vi "WS1050 16 DUT VSA-CV Sweep HD_Cycling_Ver1.3a.vi"() -> ()   [LabVIEW 2012]
uses:
  WS_VCAP Driver 024/Source/WSVCAP Shell/Type Defs/WSVCAP SHL I2C DUT Mask Mode Enum.ctl
  <vilib>/Utility/file.llb/Read From Spreadsheet File (DBL).vi
panel:
  out "VISA resource name out":refnum<visa-resource-name>="GPIB0::3::INSTR"
  out "date string":string="5/19/2014"
  out "PS1 Out":refnum<visa-resource-name>
  out "Ke2000 Out":refnum<visa-resource-name>="GPIB0::9::INSTR"
  in  "Tab Control":enum32{"Inst Control", "Data Output", "Graphs"}(tab)
  in  "Bank to HD":u16(ring)=5 items=["All OFF", "All ON", "Bank_C1", "Bank_C2", "Bank_C3", "F12+B1", "B1"]
  out "AD7747 Values":string[][](table)
  in  "Lot#":string="4NEMB"
  in  "Wafer#":string="20-EB"
  in  "File Name":string="HD_4NEMB_25_EB_65C_44V_100DC_BRD2_150916_1"
  in  "TMN DC\\CAP Data Log File Path":path=path "C:/WS1050 16 DUT Data"
  in  "SN":string[](array[string])=["1", "2", "3", "4", "5", "6", "7", "8", "9", "10", "11", "12", "13", "14", "15", "16"]
  in  "Test Program":string="WS1050 16 DUT VSA_CV Sweep HD_Cycling Ver1.3a"
  out "Current Date":string="8/28/2014"
  out "Current Time":string="0950"
  in  "Start Date":string="4/24/2014"
  in  "Start Time":string="1542"
  in  "Comment":string="CV Sweep"
  in  "OK Button":bool
  in  "Calibration":bool
  in  "Control Setting":bool
  in  "CP Setting":i32(ring) items=["CP OFF", "CP ON", "CP 35V", "CP 40V", "CP 44V", "CP 50V", "DVA OFF", "DVA ON", "Reg1 ON", "Reg1 OFF", "Reg2 ON", "Reg2 OFF", "Reg3 ON", "Reg3 OFF"]
  in  "VDD(V)":dbl=3.3 format="%.3g"
  in  "Meas Clock Rate (Hz)":dbl=1000000.0 caption="Meas Speed" format="%.1p Hz"
  out "AR  Measurent(Hz)":dbl
  in  "PS1 Source":refnum<visa-resource-name>="GPIB0::5::INSTR"
  in  "Ke2000":refnum<visa-resource-name>="GPIB0::9::INSTR"
  out "Simulate FPGA":bool
  out "Online":bool
  in  "Ke2400":refnum<visa-resource-name>="GPIB0::3::INSTR"
  in  "Initialize AD7747":bool
  in  "DUT Mask Mode":T1=enum."All"
  in  "RFFE Slave Address":u8=7 caption="Slave Address" format="0x%02x"
  out "Activity Log":string="05/19/2014 -- 12:24:35.853::WSVCAP::APP::Application Started\n05/19/2014 -- 12:24:37.606::WSVCAP::WSVCAP SHL::WR I2C-REG:0x0A;MASK:0xFFFFFFFFFFFF;C1 DATA:22:22:22:22:22:22:22:22:22:22:22:22:22:22:22:22;C2 DATA:22:22:22:22:22:22:22:22:22:22:22:22:22:22:22:22;C3 DATA:22:22:22:22:22:22:22:22:22:22:22:22:22:22:22:22\r\n05/19/2014 -- 12:24:37.773::WSVCAP::WSVCAP SHL::WR I2C-ST:0,0,4,1\r\n05/19/2014 -- 12:24:37.903::WSVCAP::WSVCAP SHL::RD I2C-BYTES:4;ADD:0x00;MASK:0xFFFFFFFFFFFF\r\n05/19/2014 -- 12:24:38.045::WSVCAP::WSVCAP SHL::RD I2C:C1 DATA:2:2:2:2:2:2:2:2:2:2:2:2:2:2:2:2|A7:A9:AA:82:82:7F:82:81:82:81:83:82:81:82:82:81|46:36:BB:88:44:A3:E9:2B:32:20:ED:25:BB:3D:68:B|2C:6A:EB:A7:22:56:FE:CC:36:82:D7:B0:3B:48:F9:CC;C2 DATA:2:2:2:2:2:2:2:2:2:2:2:2:2:2:2:2|94:94:94:80:80:80:80:80:81:7E:7E:81:80:7E:80:80|47:33:15:82:62:B:E8:1C:D7:C3:7D:41:7C:B7:4C:2A|C4:B4:AE:8:1E:D1:4E:37:11:C0:6F:63:42:9D:63:B5;C3 DATA:2:2:2:2:2:2:2:2:2:2:2:2:2:2:2:2|95:95:95:81:81:7E:81:80:84:7D:80:83:81:7E:7F:80|AB:C4:14:B5:7B:52:DF:C9:79:5D:5F:30:99:31:1E:F4|6E:5C:F7:A8:C3:EB:7B:EF:33:92:89:77:4D:67:75:DD;STATUS:0:0:4:0\r\n05/19/2014 -- 12:24:38.046::WSVCAP::WSVCAP SHL::WR I2C-REG:0x0A;MASK:0xFFFFFFFFFFFF;C1 DATA:22:22:22:22:22:22:22:22:22:22:22:22:22:22:22:22;C2 DATA:22:22:22:22:22:22:22:22:22:22:22:22:22:22:22:22;C3 DATA:22:22:22:22:22:22:22:22:22:22:22:22:22:22:22:22\r\n05/19/2014 -- 12:24:38.089::WSVCAP::WSVCAP SHL::WR I2C-ST:0,0,4,1\r\n05/19/2014 -- 12:24:38.219::WSVCAP::WSVCAP SHL::RD I2C-BYTES:4;ADD:0x00;MASK:0xFFFFFFFFFFFF\r\n05/19/2014 -- 12:24:38.362::WSVCAP::WSVCAP SHL::RD I2C:C1 DATA:2:2:2:2:2:2:2:2:2:2:2:2:2:2:2:2|A7:AB:AA:82:82:82:83:83:82:82:82:82:7F:82:82:81|4B:32:96:83:3E:61:43:17:25:62:AB:4D:A2:40:2E:5|3C:76:2B:B4:EE:E4:A9:1A:AA:A:26:C7:21:2E:87:5B;C2 DATA:2:2:2:2:2:2:2:2:2:2:2:2:2:2:2:2|94:94:94:80:80:80:80:80:80:7F:80:81:80:80:7F:80|4A:32:19:7D:19:6C:79:46:61:7F:4B:B8:A5:30:F3:14|B4:70:A:8C:9C:DC:43:FA:1E:A:C6:21:A:A9:13:F3;C3 DATA:2:2:2:2:2:2:2:2:2:2:2:2:2:2:2:2|95:97:94:81:80:81:82:81:80:7E:81:84:7F:81:80:80|B2:32:D0:A7:9E:4C:AB:D4:EE:D9:F0:82:B7:91:7:FF|C1:91:B6:3D:D8:E:1B:4F:9F:6A:F1:6C:E7:3F:7:BA;STATUS:0:0:4:0\r\n05/19/2014 -- 12:24:38.364::WSVCAP::WSVCAP SHL::WR I2C-REG:0x0A;MASK:0xFFFFFFFFFFFF;C1 DATA:22:22:22:22:22:22:22:22:22:22:22:22:22:22:22:22;C2 DATA:22:22:22:22:22:22:22:22:22:22:22:22:22:22:22:22;C3 DATA:22:22:22:22:22:22:22:22:22:22:22:22:22:22:22:22\r\n05/19/2014 -- 12:24:38.406::WSVCAP::WSVCAP SHL::WR I2C-ST:0,0,4,1\r\n05/19/2014 -- 12:24:38.536::WSVCAP::WSVCAP SHL::RD I2C-BYTES:4;ADD:0x00;MASK:0xFFFFFFFFFFFF\r\n05/19/2014 -- 12:24:38.678::WSVCAP::WSVCAP SHL::RD I2C:C1 DATA:2:2:2:2:2:2:2:2:2:2:2:2:2:2:2:2|A7:A9:AB:82:82:81:82:82:82:82:82:82:82:82:82:81|46:71:4C:87:43:3D:7F:FC:25:4F:8E:54:97:3E:60:8C|AA:F4:1F:B5:CE:43:1F:36:9:87:9C:78:86:5:B6:8E;C2 DATA:2:2:2:2:2:2:2:2:2:2:2:2:2:2:2:2|94:94:94:80:7F:7F:80:80:80:80:80:81:80:80:80:80|49:36:18:7D:6E:C5:E4:3C:81:2E:41:D3:75:71:E3:72|E8:D3:E6:D1:E0:48:AE:D4:54:D:E8:8E:B4:41:68:4;C3 DATA:2:2:2:2:2:2:2:2:2:2:2:2:2:2:2:2|95:95:95:81:7F:7F:81:81:81:81:81:84:81:81:82:81|B3:F5:90:AB:82:69:7B:93:D0:77:E8:D5:E8:8C:84:E8|B9:AC:EE:2B:B6:71:8F:4A:74:31:56:BB:8A:B7:A0:C8;STATUS:0:0:4:0\r\n05/19/2014 -- 12:24:38.681::WSVCAP::WSVCAP SHL::WR I2C-REG:0x0A;MASK:0xFFFFFFFFFFFF;C1 DATA:22:22:22:22:22:22:22:22:22:22:22:22:22:22:22:22;C2 DATA:22:22:22:22:22:22:22:22:22:22:22:22:22:22:22:22;C3 DATA:22:22:22:22:22:22:22:22:22:22:22:22:22:22:22:22\r\n05/19/2014 -- 12:24:38.723::WSVCAP::WSVCAP SHL::WR I2C-ST:0,0,4,1\r\n05/19/2014 -- 12:24:38.854::WSVCAP::WSVCAP SHL::RD I2C-BYTES:4;ADD:0x00;MASK:0xFFFFFFFFFFFF\r\n05/19/2014 -- 12:24:38.996::WSVCAP::WSVCAP SHL::RD I2C:C1 DATA:2:2:2:2:2:2:2:2:2:2:2:2:2:2:2:2|A7:A9:AA:82:82:7F:83:81:82:81:84:82:7F:82:7F:82|43:FB:E:7F:3C:AD:35:35:26:A2:6C:21:4B:3D:8:6|63:9A:E1:F3:95:32:91:42:90:3C:78:1F:5C:D7:5F:D8;C2 DATA:2:2:2:2:2:2:2:2:2:2:2:2:2:2:2:2|94:94:94:80:80:80:80:80:81:80:7E:81:80:7E:7F:80|48:36:18:7F:5E:3D:69:83:DE:AE:A1:9E:31:AE:BB:96|15:A0:44:17:13:FD:CC:C8:6D:B2:EF:A7:C:C7:3B:F;C3 DATA:2:2:2:2:2:2:2:2:2:2:2:2:2:2:2:2|95:96:94:81:81:7E:82:80:84:80:80:84:7F:7E:7D:82|AD:3B:6D:A9:7C:57:9D:F5:7A:96:23:5C:36:2D:ED:5A|CD:46:DB:3B:C7:BD:70:60:33:B8:B:F7:63:A:51:4D;STATUS:0:0:4:0\r\n05/19/2014 -- 12:24:38.998::WSVCAP::WSVCAP SHL::WR I2C-REG:0x0A;MASK:0xFFFFFFFFFFFF;C1 DATA:22:22:22:22:22:22:22:22:22:22:22:22:22:22:22:22;C2 DATA:22:22:22:22:22:22:22:22:22:22:22:22:22:22:22:22;C3 DATA:22:22:22:22:22:22:22:22:22:22:22:22:22:22:22:22\r\n05/19/2014 -- 12:24:39.040::WSVCAP::WSVCAP SHL::WR I2C-ST:0,0,4,1\r\n05/19/2014 -- 12:24:39.170::WSVCAP::WSVCAP SHL::RD I2C-BYTES:4;ADD:0x00;MASK:0xFFFFFFFFFFFF\r\n05/19/2014 -- 12:24:39.311::WSVCAP::WSVCAP SHL::RD I2C:C1 DATA:2:2:2:2:2:2:2:2:2:2:2:2:2:2:2:2|A7:AA:AB:82:82:81:82:81:82:81:82:82:82:82:7F:82|44:F1:90:87:45:44:C8:2C:2C:F1:FC:1B:94:3B:3C:75|4A:49:95:19:99:73:64:3:23:24:F3:A2:5E:7F:C4:B6;C2 DATA:2:2:2:2:2:2:2:2:2:2:2:2:2:2:2:2|94:94:94:80:80:80:80:7F:80:80:7E:80:80:7E:7F:80|4C:36:17:7D:A8:9F:DE:C7:53:6D:8A:F4:41:A5:C6:E0|90:2E:24:C:D9:22:E4:76:3B:40:1D:53:33:B1:3E:4D;C3 DATA:2:2:2:2:2:2:2:2:2:2:2:2:2:2:2:2|95:97:95:81:81:7F:81:80:80:81:7F:82:81:7E:7D:82|AE:2B:A7:AB:CC:CD:A4:38:FD:17:80:F2:92:2D:45:C4|76:E5:D:B9:AD:B5:BA:8D:28:32:9E:42:B7:20:4A:D9;STATUS:0:0:4:0\r\n05/19/2014 -- 12:24:39.313::WSVCAP::WSVCAP SHL::WR I2C-REG:0x0A;MASK:0xFFFFFFFFFFFF;C1 DATA:22:22:22:22:22:22:22:22:22:22:22:22:22:22:22:22;C2 DATA:22:22:22:22:22:22:22:22:22:22:22:22:22:22:22:22;C3 DATA:22:22:22:22:22:22:22:22:22:22:22:22:22:22:22:22\r\n05/19/2014 -- 12:24:39.355::WSVCAP::WSVCAP SHL::WR I2C-ST:0,0,4,1\r\n05/19/2014 -- 12:24:39.486::WSVCAP::WSVCAP SHL::RD I2C-BYTES:4;ADD:0x00;MASK:0xFFFFFFFFFFFF\r\n05/19/2014 -- 12:24:39.628::WSVCAP::WSVCAP SHL::RD I2C:C1 DATA:2:2:2:2:2:2:2:2:2:2:2:2:2:2:2:2|A7:A9:AA:82:82:82:83:82:82:82:82:82:7F:82:7F:82|47:18:E4:87:3E:E7:6:65:25:92:37:38:A8:3E:89:85|7C:A7:7:2B:A3:7A:EC:EF:89:ED:F4:D3:D8:BC:3A:F5;C2 DATA:2:2:2:2:2:2:2:2:2:2:2:2:2:2:2:2|94:94:94:80:7F:80:80:7F:81:80:7E:80:80:80:81:80|49:37:17:80:76:25:6A:F8:DF:55:97:4D:B8:5B:2B:B1|13:E3:9A:3E:1A:2D:4F:B6:DB:E9:61:FA:8B:D6:9:CC;C3 DATA:2:2:2:2:2:2:2:2:2:2:2:2:2:2:2:2|95:95:95:81:7F:80:82:81:84:80:7F:81:80:81:7F:82|AF:93:3B:AF:5B:11:82:E4:7E:C3:2D:72:9:96:D9:A|DB:96:F2:10:5F:64:9A:C6:98:12:27:7D:10:D3:20:D9;STATUS:0:0:4:0\r\n05/19/2014 -- 12:24:40.132::WSVCAP::WSVCAP SHL::CLOSE\r\n"
  in  "C1 Cap DAC":u8=128 caption="B Data In" format="0x%02x"
  in  "C2 Cap DAC":u8=128 caption="B Data In" format="0x%02x"
  in  "C3 Cap DAC":u8=128 caption="B Data In" format="0x%02x"
  out "IDD Brd(uA)":string
  in  "VSA_IDD(A)":dbl=0.1
  in  "Stress Voltage(V)":dbl
  in  "Reset PS":bool
  in  "HD/Cycling":bool
  in  "Cyc Clock Rate (Hz)":dbl=5000000.0 caption="Cycle Speed" format="%.1p Hz"
  in  "Bank to Cycle":u16(ring)=1 items=["Cycle All", "Cycle F12+S1", "Cycle All - F12"]
  in  "Set Delay":dbl[](array[numeric])=[1.8e-05, 1.8e-05, 1.8e-05] min=0.0 max=0.5 format="%#.0p s"
  in  "CP Freq":u16(ring)=3 items=["000", "001", "010", "011", "100", "101", "110", "111"]
  in  "CP to HD/Cycle":i32(ring)=4 items=["CP HDC 35V", "CP HDC 40.25V", "CP HDC 27.5V", "CP HDC 30.5V", "CP HDC 44V", "CP HDC 50V"]
  in  "Cycle Freq(KHz)":dbl
  in  "RP will be\nFrom Lookup Table":bool
  in  "Keep B1 Close?":bool
  out "STATUS":string="Idle...."
  in  "stop":bool
  out "C1 Min_T0":string[](array[string])
  out "CAP_Value(pF)":string[][](array[string])
  out "C3 Min_T0":string[](array[string])
  out "C2 Min_T0":string[](array[string])
  in  "Abort":bool
  out "error out 2":errorcluster
  in  "Set Stress to\nComplete(Cyc/Min)":u64=8100
  out "Verify Test Condition":string[](array[string])
  out "CMin+VCAP":string[][](table)
  out "Verify Drivers to Stress":string[](array[string])
  out "Cycle Count":u64 min=1 max=4 step=1
  out "Stress \nCompleted(Min)":u64
  out "Previous Time":string="12:20:26 PM"
  out "Delta CAP_T0(pF)":dbl[][](array[numeric])
  out "Delta CAP_Tc(pF)":dbl[][](array[numeric])
  in  "error in (no error)":errorcluster
  out "error out":errorcluster
  out "CP_IDD(uA)":string
  # "Company:  WiSpry Inc 20 Fairbanks \nSte 198 Irvine CA 92618\n\nAuthor:  Andy V Tran\nCreated:  02/10/2016\nLabVIEW 2012 Pro\nTP:  WS1050 16 DUT VSA_CV Sweep HD_Cycling Ver1.3a\nFPGA Version: WS_VCAP Driver 024"
  # "Note:  Ver1.0 is a original version.\n\n1.  Two look up tables, \n      a.  1st is for Stress\n      b.  2nd is for Voltage sweep\n\nVer1.1\n\n1.  No Voltage to CAP Head for initial read point\n\nVer1.2\n\n1.  Add CP Freq\n\nVer1.3\n\n1.  Add Cycling Stress\n2.  Add a button for Readpoint from look up table\n3.  Add a selectable drivers for HD\n\nSet up and Test Sequences:\n\n1.  Calibration with Empty Sockets\n2.  Load Parts\n3.  Set condition to stress (CP Voltage, Drivers to Stress, CP to stress...)\n4.  Set Date/Time to start stressing\n5.  Set TTF to stop stressing (default = 135 hrs)"
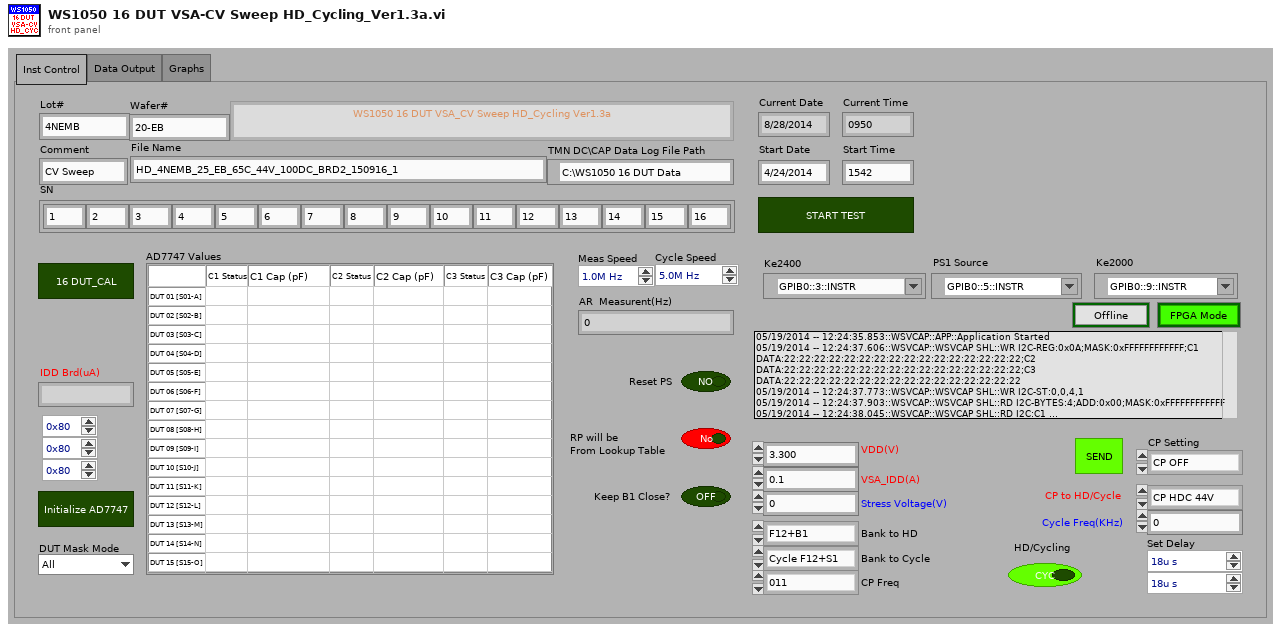
[diagram p1: front panel]
types:
  T1 = typedef "WSVCAP SHL I2C DUT Mask Mode Enum.ctl" = enum16{"Custom", "C1", "C2", "C3", "All"}
  T2 = typedef "WSVCAP SHL Core System Cluster.ctl" = cluster{"Settings":T3, "FPGA Resource":tag, "Online":bool, "I2C Wait Ticks":u32, "SPI Wait Ticks":u32, "RFFE Wait Ticks":u32}
  T3 = typedef "WSVCAP SHL I2C Settings Cluster.ctl" = cluster{"FPGA Resource Name":string, "I2C Slave Address":u8, "I2C Clock Rate (Hz)":dbl, "SPI Clock Rate (Hz)":dbl, "RFFE Slave Address":u8, "RFFE Clock Rate (Hz)":dbl, "Simulate FPGA":bool, "C1 Cap DAC Default":u8, "C2 Cap DAC Default":u8, "C3 Cap DAC Default":u8}
  T4 = enum16{"Idle...", "Voltage 1", "Voltage 2", "Voltage 3"}[]
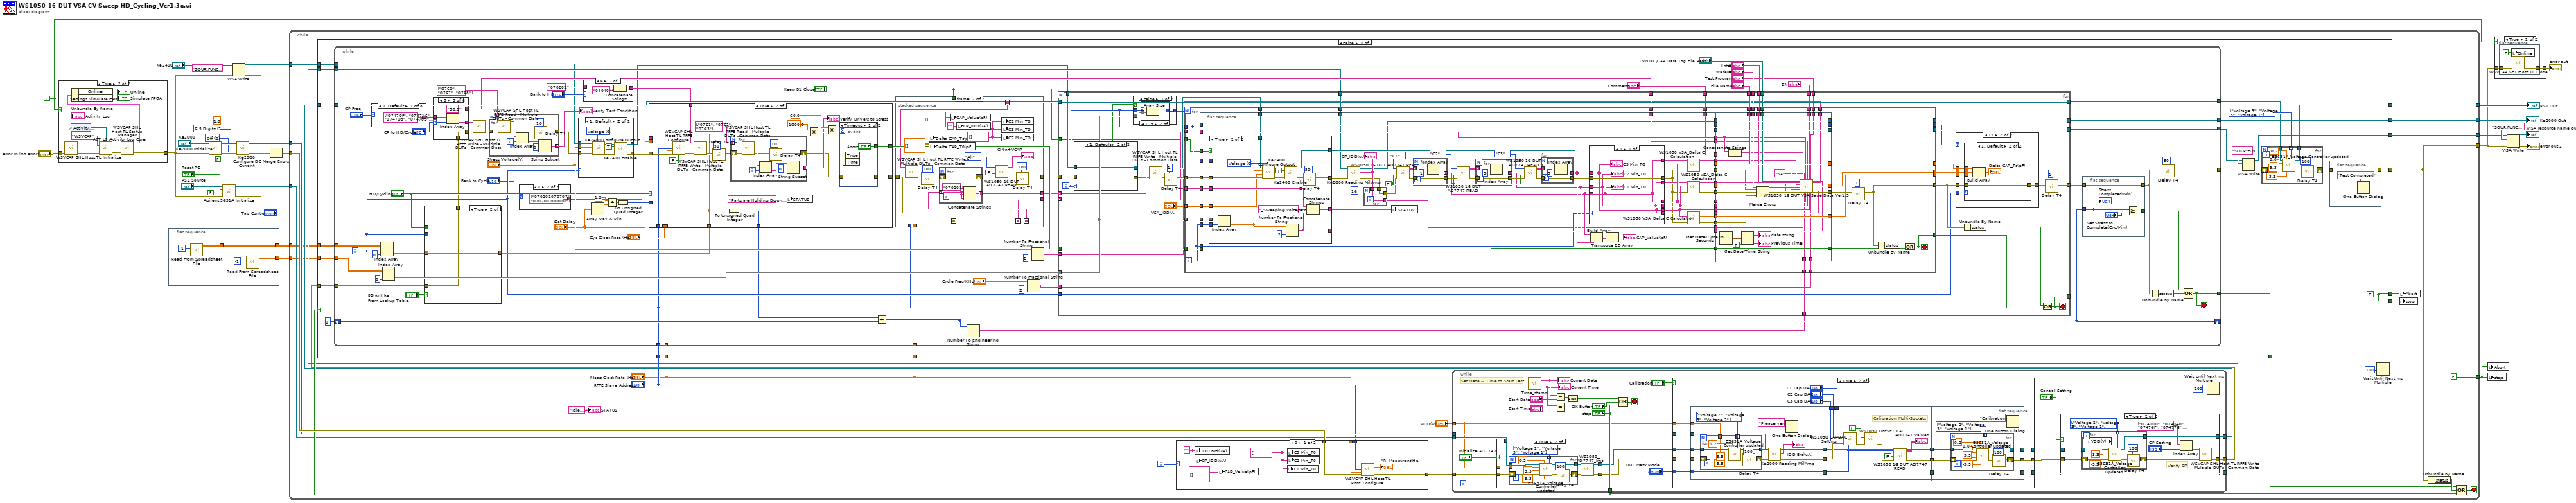
[diagram p0: block diagram]
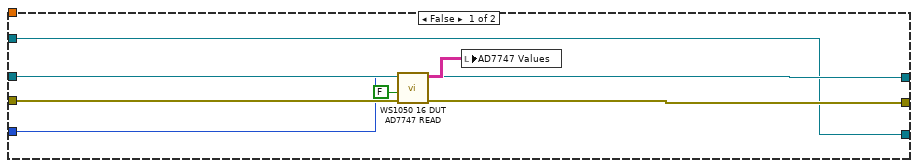
[diagram p7: hidden frame]
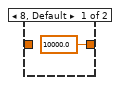
[diagram p9: hidden frame]
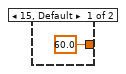
[diagram p11: hidden frame]
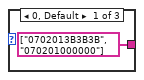
[diagram p12: hidden frame]
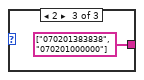
[diagram p13: hidden frame]
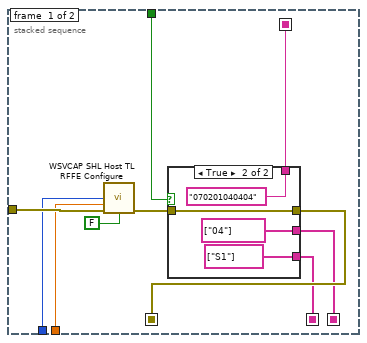
[diagram p14: hidden frame]
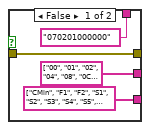
[diagram p15: hidden frame]
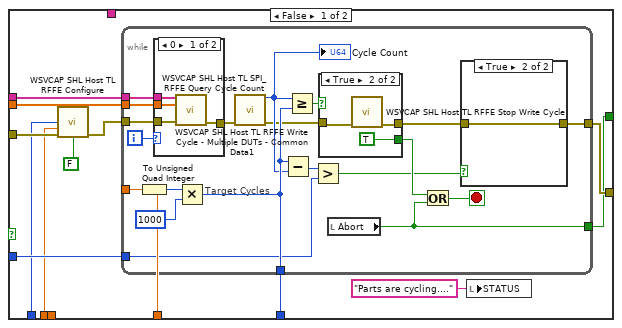
[diagram p16: hidden frame]
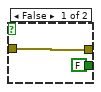
[diagram p19: hidden frame]
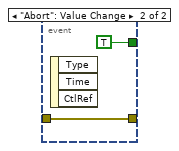
[diagram p20: hidden frame]
diagram:
  w21 = TRUE
  w27 = u16 0 items=["Off", "Moving Filter", "Repeating Filter"] ("Digital Filter (0: Off)")
  w28 = u16 7 items=["3.5 Digits"=4, "4.5 Digits"=5, "5.5 Digits"=6, "6.5 Digits"=7] ("Resolution (7: 6.5 digits)")
  n1 = case shown="True" w21 {
    tunnel: "error in (no error)" -> [w35 w36]
    tunnel: [w35 w43] -> w10
    frame False {
    }
    frame True {
      n2 = call "WSVCAP SHL Host TL Initialize.vi"("error in"=w36) -> ("error out"=w37:errorcluster)  [unwired: 13 in, 1 out]
      n3 = control-ref of="Activity Log"() -> (w39:refnum<vi>)
      n4 = call "ACT LG Activity Log Core.vi"("Display Ref"=w39, "Source"="WSVCAP", "Error In (no error)"=w37) -> ("Error Out"=w38:errorcluster)  [unwired: 11 in, 1 out]
      n5 = call "WSVCAP SHL Host TL Status Manager.vi"("error in"=w38) -> ("System Out"=w44:T2, "error out"=w43:errorcluster)  [unwired: 13 in]
      n6 = Unbundle By Name(w44) -> ("Online"=→"Online":bool, "Settings.Simulate FPGA"=→"Simulate FPGA":bool)
    }
  }
  n7 = flat-sequence {
    tunnel: [w46] -> w5
    tunnel: w5 -> [w49]
    tunnel: [w49] -> w4
    tunnel: [w48] -> w3
    frame #0 {
      n8 = call-poly <vilib>:"Read From Spreadsheet File.vi"("number of rows (all:-1)"=-1) -> ("all rows"=w46:dbl[][])  [unwired: 6 in, 4 out]
    }
    frame #1 {
      n9 = call-poly <vilib>:"Read From Spreadsheet File.vi"("number of rows (all:-1)"=-1) -> ("all rows"=w48:dbl[][])  [unwired: 6 in, 4 out]
    }
  }
  n10 = call "Ke2000 Initialize.vi"("error in (no error)"=w10, "VISA resource name"="Ke2000") -> ("error out"=w29:errorcluster, "VISA resource name out"=w30:refnum<visa-resource-name>)  [unwired: 8 in]
  n11 = call "Agilent 3631A Initialize.vi"("error in (no error)"=w10, "Default"=FALSE ("Reset? (T: Yes)"), "Reset"="Reset PS", "VISA resource name"="PS1 Source") -> ("error out"=w9:errorcluster, "VISA resource name out"=w33:refnum<visa-resource-name>)  [unwired: 6 in]
  n12 = VISA Write(VISA resource name="Ke2400", write buffer="SOUR:FUNC VOLT;VOLT:MODE FIX;RANG 100;LEV 0.0;:SENS:FUNC \"CURR\";CURR:PROT 60E-3;RANG 100E-3;:OUTP ON", error in (no error)=w10) -> (VISA resource name out=w18:refnum<visa-resource-name>, error out=w13:errorcluster)  [unwired: 1 out]
  n13 = call "Ke2000 Configure DC Current.vi"("Resolution (7: 6.5 digits)"=w28, "Digital Filter (0: Off)"=w27, "Auto Range? (T: Auto)"=FALSE, "error in"=w29, "Custom Range (0 A)"=1.0, "VISA resource name"=w30) -> ("error out"=w11:errorcluster, "VISA resource name out"=w25:refnum<visa-resource-name>)  [unwired: 4 in]
  n14 = Merge Errors(w13, w11, w9) -> (w19:errorcluster)
  n15 = while {
    tunnel: w19 -> [w70]
    tunnel: [w60] -> w15
    tunnel: w33 -> [w64]
    tunnel: w25 -> [w65]
    tunnel: [w73] -> w24
    tunnel: [w72] -> w23
    tunnel: w18 -> [w69]
    tunnel: [w68] -> w16
    tunnel: [FALSE] -> w8
    tunnel: w4 -> [w56]
    tunnel: w3 -> [w55]
    i -> [w71]
    stop <- w74 stop-if-true
    n16 = case shown="0" w71 {
      tunnel: w70 -> [w84 w85]
      tunnel: [w83 w85] -> w66
      tunnel: "RFFE Slave Address" -> [w81 _]
      tunnel: "Meas Clock Rate (Hz)" -> [w77 _]
      frame 0 {
        w80 = string[] []
        w78 = "" ("uA")
        n17 = local write "IDD Brd(uA)"(w78) -> ()
        n18 = local write "CP_IDD(uA)"(w78) -> ()
        n19 = local write "CAP_Value(pF)"(string[][] []) -> ()
        n20 = local write "C1 Min_T0"(w80) -> ()
        n21 = local write "C3 Min_T0"(w80) -> ()
        n22 = local write "C2 Min_T0"(w80) -> ()
        n23 = call "WSVCAP SHL Host TL RFFE Configure.vi"("RFFE Slave Address"=w81, "Clock Rate (Hz)"=w77, "error in"=w84) -> ("Actual Rate (Hz)"=→"AR  Measurent(Hz)":dbl, "error out"=w83:errorcluster)  [unwired: 11 in]
      }
      frame 1, Default {
      }
    }
    n24 = while {
      tunnel: ["stop"] -> w67
      tunnel: w66 -> [w97]
      tunnel: [w89] -> w61
      tunnel: w64 -> [w95]
      tunnel: w65 -> [w91]
      tunnel: [w92] -> w63
      tunnel: [w90] -> w62
      tunnel: "VDD(V)" -> [w87]
      stop <- w104 stop-if-true
      # "Set Date & Time to Start Test"
      n25 = case shown="True" "Initialize AD7747" {
        tunnel: w97 -> [w113 w119]
        tunnel: [w113 w115] -> w96
        tunnel: w95 -> [w112 w117]
        tunnel: [w112 w116] -> w94
        tunnel: w87 -> [_ w114]
        frame False {
        }
        frame True {
          w120 = T4 [enum."Voltage 2", enum."Voltage 3", enum."Voltage 1"] items=["Idle...", "Voltage 1", "Voltage 2", "Voltage 3"]
          n26 = for {
            tunnel: w117 -> [w130]
            tunnel: w120 -> [w128] mode=indexing
            tunnel: [w127] -> w116
            shift-right: [w124] -> w118
            shift-left: w119 -> [w131]
            tunnel: w114 -> [w122]
            n27 = call "E3631A_Voltage Controller updated.vi"("VISA resource name"=w130, "I_VDD(A)"=0.2, "Channel Controller"=w128, "Voltage 1"=w122, "Voltage 2"=3.3, "error in (no error)"=w131, "Voltage 3"=-3.3) -> ("VISA resource name out"=w127:refnum<visa-resource-name>, "error out"=w123:errorcluster)  [unwired: 7 in]
            n28 = call "Delay T4.vi"("milliseconds to wait"=u32 100, "error in (no error)"=w123) -> ("error out"=w124:errorcluster)  [unwired: 9 in]
          }
          n29 = call "WS1050_AD7747_Init.vi"("error in"=w118) -> ("error out"=w115:errorcluster)  [unwired: 10 in]
        }
      }
      n30 = call "Time_stamp.vi"() -> ("date/time string"=w109:string, "date string"=w111:string)  [unwired: 2 in]
      "Current Date" <- w111
      "Current Time" <- w109
      n31 = Equal?(x=w111, y="Start Date") -> (x = y?=w107:bool)
      n32 = Equal?(x=w109, y="Start Time") -> (x = y?=w106:bool)
      n33 = And(x=w107, y=w106) -> (x .and. y?=w103:bool)
      n34 = Compound Arithmetic op=OR(w103, "OK Button", "stop") -> (w104:bool)
      n35 = case shown="True" "Calibration" {
        tunnel: w96 -> [w158 w177]
        tunnel: [w157 w174] -> w88
        tunnel: w94 -> [w156 w173]
        tunnel: "DUT Mask Mode" -> [w155 w169]
        tunnel: [w156 w168] -> w93
        tunnel: w91 -> [w154 w164]
        tunnel: [w154 w161] -> w90
        tunnel: w87 -> [_ w160]
        frame False {
          n36 = call "WS1050 16 DUT AD7747 READ.vi"("error in"=w158, "Log (T)"=FALSE, "DUT Mask Mode (All)"=w155) -> ("error out"=w157:errorcluster, "AD7747 Values"=w159:string[][])  [unwired: 7 in]
          n37 = local write "AD7747 Values"(w159) -> ()
        }
        frame True {
          n38 = flat-sequence {
            tunnel: w177 -> [w187]
            tunnel: [w182] -> w176
            tunnel: w173 -> [w186]
            tunnel: [w185] -> w172
            tunnel: w169 -> [w184]
            tunnel: [w184] -> w170
            tunnel: w164 -> [w180]
            tunnel: [w179] -> w163
            tunnel: w160 -> [w178]
            tunnel: w176 -> [w213]
            tunnel: [w212] -> w175
            tunnel: w172 -> [w211]
            tunnel: [w211] -> w171
            tunnel: w170 -> [w210]
            tunnel: "C1 Cap DAC" -> [w206]
            tunnel: "C2 Cap DAC" -> [w205]
            tunnel: "C3 Cap DAC" -> [w204]
            tunnel: w163 -> [w203]
            tunnel: [w203] -> w162
            tunnel: w175 -> [w216]
            tunnel: [w219] -> w174
            tunnel: w171 -> [w218]
            tunnel: [w215] -> w168
            tunnel: w162 -> [w214]
            tunnel: [w214] -> w161
            frame #0 {
              w188 = T4 [enum."Voltage 2", enum."Voltage 3", enum."Voltage 2"] items=["Idle...", "Voltage 1", "Voltage 2", "Voltage 3"]
              n39 = for {
                tunnel: w186 -> [w199]
                tunnel: w188 -> [w196] mode=indexing
                tunnel: [w195] -> w185
                shift-right: [w193] -> w181
                shift-left: w187 -> [w200]
                tunnel: w178 -> [w190]
                n40 = call "E3631A_Voltage Controller updated.vi"("VISA resource name"=w199, "I_VDD(A)"=0.2, "Channel Controller"=w196, "Voltage 1"=w190, "Voltage 2"=3.3, "error in (no error)"=w200, "Voltage 3"=-3.3) -> ("VISA resource name out"=w195:refnum<visa-resource-name>, "error out"=w192:errorcluster)  [unwired: 7 in]
                n41 = call "Delay T4.vi"("milliseconds to wait"=u32 100, "error in (no error)"=w192) -> ("error out"=w193:errorcluster)  [unwired: 9 in]
              }
              n42 = call "Ke2000 Reading MilAmp.vi"("error in (no error)"=w181, "VISA resource name"=w180) -> ("error out"=w182:errorcluster, "uA"=→"IDD Brd(uA)":string, "VISA resource name out"=w179:refnum<visa-resource-name>)  [unwired: 7 in]
              n43 = One Button Dialog(message="Please verify all sockets should be empty...") -> ()  [unwired: 1 in, 1 out]
            }
            frame #1 {
              # "Calibration Multi-Sockets"
              n44 = call "WS1050 CAPDAC Setting.vi"("DUT Mask Mode (All)"=w210, "error in"=w213, "C3 Cap DAC"=w204, "C2 Cap DAC"=w205, "C1 Cap DAC"=w206) -> ("error out"=w208:errorcluster)  [unwired: 5 in, 1 out]
              n45 = call "WS1050 OFFSET CAL.vi"("error in"=w208, "OFFSET CAL"=TRUE ("Read?")) -> ("error out"=w207:errorcluster)  [unwired: 8 in, 1 out]
              n46 = call "WS1050 16 DUT AD7747 READ.vi"("error in"=w207, "Log (T)"=FALSE, "DUT Mask Mode (All)"=w210) -> ("error out"=w212:errorcluster, "AD7747 Values"=→"AD7747 Values":string[][])  [unwired: 7 in]
            }
            frame #2 {
              w217 = T4 [enum."Voltage 2", enum."Voltage 3", enum."Voltage 1"] items=["Idle...", "Voltage 1", "Voltage 2", "Voltage 3"]
              n47 = for {
                tunnel: w218 -> [w231]
                tunnel: w217 -> [w227] mode=indexing
                tunnel: [w226] -> w215
                shift-right: [w222] -> w219
                shift-left: w216 -> [w228]
                n48 = call "E3631A_Voltage Controller updated.vi"("VISA resource name"=w231, "I_VDD(A)"=0.2, "Channel Controller"=w227, "Voltage 1"=0.0, "Voltage 2"=3.3, "error in (no error)"=w228, "Voltage 3"=-3.3) -> ("VISA resource name out"=w226:refnum<visa-resource-name>, "error out"=w221:errorcluster)  [unwired: 7 in]
                n49 = call "Delay T4.vi"("milliseconds to wait"=u32 100, "error in (no error)"=w221) -> ("error out"=w222:errorcluster)  [unwired: 9 in]
              }
              n50 = One Button Dialog(message="Calibration Completed....") -> ()  [unwired: 1 in, 1 out]
            }
          }
        }
      }
      n51 = case shown="True" "Control Setting" {
        tunnel: [w132 w135] -> w89
        tunnel: w93 -> [w133 w138]
        tunnel: [w133 w136] -> w92
        tunnel: w88 -> [w132 w134]
        frame False {
        }
        frame True {
          w139 = T4 [enum."Voltage 2", enum."Voltage 3", enum."Voltage 1"] items=["Idle...", "Voltage 1", "Voltage 2", "Voltage 3"]
          # "Verify CP"
          n52 = for {
            tunnel: w138 -> [w151]
            tunnel: w139 -> [w148] mode=indexing
            shift-right: [w145] -> w137
            shift-left: w134 -> [w152]
            tunnel: [w143] -> w136
            n53 = local read "VDD(V)"() -> (w147:dbl)
            n54 = call "E3631A_Voltage Controller updated.vi"("VISA resource name"=w151, "Channel Controller"=w148, "Voltage 1"=w147, "Voltage 2"=3.3, "error in (no error)"=w152, "Voltage 3"=-3.3) -> ("VISA resource name out"=w143:refnum<visa-resource-name>, "error out"=w146:errorcluster)  [unwired: 8 in]
            n55 = call "Delay T4.vi"("milliseconds to wait"=u32 100, "error in (no error)"=w146) -> ("error out"=w145:errorcluster)  [unwired: 9 in]
          }
          n56 = Index Array(array=string[] ["074000", "074040", "07476F", "074776", "07477B", "07477C", "074820", "074800", "07413B", "074100", "07423B", "074200", "07433B", "074300"], index="CP Setting") -> (element=w140:string)
          n57 = call "WSVCAP SHL Host TL RFFE Write - Multiple DUTs - Common Data.vi"("Data Out"=w140, "error in"=w137) -> ("error out"=w135:errorcluster)  [unwired: 13 in]
        }
      }
      n58 = Wait Until Next ms Multiple(millisecond multiple=u32 100) -> ()  [unwired: 1 out]
    }
    n59 = case shown="False" w67 {
      tunnel: w61 -> [w251 w887]
      tunnel: [w235 w887] -> w60
      tunnel: w63 -> [w249 w885]
      tunnel: w62 -> [w252 w886]
      tunnel: [w248 w886] -> w73
      tunnel: [w239 w885] -> w72
      tunnel: w69 -> [w254 w884]
      tunnel: [w250 w884] -> w68
      tunnel: [w247 w883] -> w58
      tunnel: [w247 w883] -> w57
      tunnel: w56 -> [w245 _]
      tunnel: w55 -> [w243 _]
      tunnel: [w238 w883] -> w53
      tunnel: "RFFE Slave Address" -> [w234 _]
      tunnel: "Meas Clock Rate (Hz)" -> [w233 _]
      tunnel: "Meas Clock Rate (Hz)" -> [w232 _]
      frame False {
        w242 = T4 [enum."Voltage 3", enum."Voltage 3", enum."Voltage 1"] items=["Idle...", "Voltage 1", "Voltage 2", "Voltage 3"]
        w247 = FALSE
        n60 = while {
          tunnel: w254 -> [w291]
          tunnel: w252 -> [w302]
          tunnel: w251 -> [w281]
          tunnel: w249 -> [w335]
          tunnel: [w334] -> w248
          tunnel: [w333] -> w240
          tunnel: [w332] -> w246
          tunnel: [w331] -> w237
          tunnel: w245 -> [w323]
          shift-right: [w316] -> _
          shift-left: u64 0 ("disabled index (col)") -> [w321]
          tunnel: w243 -> [w314]
          tunnel: [w299] -> w238
          tunnel: w234 -> [w276]
          tunnel: w233 -> [w279]
          tunnel: w232 -> [w275]
          i -> [w282]
          stop <- w299 stop-if-true
          n61 = case shown="0, Default" "CP Freq" {
            tunnel: [string[] ["07470F", "074716", "074705", "074709", "07471B", "07471C"] string[] ["07471F", "074736", "074715", "074719", "07473B", "07473C"] string[] ["07474F", "074756", "074745", "074749", "07475B", "07475C"] string[] ["07476F", "074776", "074765", "074769", "07477B", "07477C"] string[] ["07478F", "074796", "074785", "074789", "07479B", "07479C"] string[] ["0747AF", "0747B6", "0747A5", "0747A9", "0747BB", "0747BC"] string[] ["0747BF", "0747C6", "0747B5", "0747B9", "0747CB", "0747CC"] string[] ["0747EF", "0747F6", "0747E5", "0747E9", "0747FB", "0747FC"]] -> w295
            frame 0, Default {
            }
            frame 1 {
            }
            frame 2 {
            }
            frame 3 {
            }
            frame 4 {
            }
            frame 5 {
            }
            frame 6 {
            }
            frame 7 {
            }
          }
          n62 = Index Array(array=w323, index (row)=w282, index (col)=0 ("disabled index (col)")) -> (element=w305:dbl)
          n63 = Index Array(array=w314, index (col)=0 ("disabled index (col)")) -> (element=w313:dbl[])  [unwired: 1 in]
          n64 = case shown="True" "RP will be\nFrom Lookup Table" {
            tunnel: w305 -> [w346 w360]
            tunnel: [w345 w360] -> w304
            tunnel: "HD/Cycling" -> [w344 _]
            tunnel: w282 -> [w343 _]
            tunnel: w281 -> [w342 w359]
            tunnel: [w341 w359] -> w280
            frame False {
              n65 = case shown="False" w344 {
                tunnel: w346 -> [w349 w356]
                tunnel: [w350 w355] -> w345
                tunnel: w343 -> [w348 w354]
                tunnel: w342 -> [w347 w353]
                tunnel: [w347 w353] -> w341
                frame False {
                  n66 = case shown="0..7" w348 {
                    tunnel: w349 -> [_ w352]
                    tunnel: [10000.0 w352] -> w350
                    frame 8, Default {
                    }
                    frame 0..7 {
                    }
                  }
                }
                frame True {
                  n67 = case shown="0..14" w354 {
                    tunnel: w356 -> [_ w358]
                    tunnel: [60.0 w358] -> w355
                    frame 15, Default {
                    }
                    frame 0..14 {
                    }
                  }
                }
              }
            }
            frame True {
            }
          }
          n68 = case shown="5" "CP to HD/Cycle" {
            selector: "CP to HD/Cycle" -> [w542 w547 w552 w557 w562 w566]
            tunnel: w295 -> [w543 w548 w553 w558 w563 w568]
            tunnel: [w541 w546 w551 w556 w561 w567] -> w328
            tunnel: ["35.0" ("Data Out") "27.5" ("Data Out") "30.5" ("Data Out") "44.0" ("Data Out") "50.0" ("Data Out") "40.25" ("Data Out")] -> w309
            tunnel: [w539 w544 w549 w554 w559 w564] -> w327
            tunnel: w280 -> [w539 w544 w549 w554 w559 w564]
            frame 0, Default {
              n69 = Index Array(array=w543, index=w542) -> (element=w541:string)
            }
            frame 2 {
              n70 = Index Array(array=w548, index=w547) -> (element=w546:string)
            }
            frame 3 {
              n71 = Index Array(array=w553, index=w552) -> (element=w551:string)
            }
            frame 4 {
              n72 = Index Array(array=w558, index=w557) -> (element=w556:string)
            }
            frame 5 {
              n73 = Index Array(array=w563, index=w562) -> (element=w561:string)
            }
            frame 1 {
              n74 = Index Array(array=w568, index=w566) -> (element=w567:string)
            }
          }
          n75 = call "WSVCAP SHL Host TL RFFE Write - Multiple DUTs - Common Data.vi"("Data Out"=w328, "error in"=w327) -> ("error out"=w325:errorcluster)  [unwired: 13 in]
          n76 = for {
            tunnel: string[] ["0760", "0767", "0768"] -> [w538] mode=indexing
            tunnel: [w534] -> w324 mode=indexing
            tunnel: w325 -> [w532]
            tunnel: [w530] -> w292
            i -> [w537]
            n77 = call "WSVCAP SHL Host TL RFFE Read - Multiple DUTs - Common Data.vi"("Data Out"=w538, "error in"=w532) -> ("RFFE Data In"=w536:string[], "error out"=w529:errorcluster)  [unwired: 12 in]
            n78 = Index Array(array=w536, index=w537) -> (element=w533:string)
            n79 = call "Delay T4.vi"("milliseconds to wait"=u32 10, "error in (no error)"=w529) -> ("error out"=w530:errorcluster)  [unwired: 9 in]
            n80 = String Subset(string=w533, offset (0)=0) -> (substring=w534:string)  [unwired: 1 in]
          }
          "Verify Test Condition" <- w324
          n81 = case shown="1" "Bank to Cycle" {
            tunnel: [string[] ["0702013B3B3B", "070201000000"] ("Command 2") string[] ["070201070707", "070201000000"] ("Command 2") string[] ["070201383838", "070201000000"] ("Command 2")] -> w273
            frame 0, Default {
            }
            frame 1 {
            }
            frame 2 {
            }
          }
          n82 = case shown="1, Default" w282 {
            tunnel: [w485 w492] -> w289
            tunnel: w292 -> [w485 w491]
            tunnel: w291 -> [w486 w490]
            tunnel: [w486 w489] -> w290
            tunnel: "Stress Voltage(V)" -> [_ w487]
            frame 0 {
            }
            frame 1, Default {
              w488 = u16 0 items=["Voltage", "Current"] ("Source Mode  (0: Voltage)")
              n83 = call "Ke2400 Configure Output.vi"("Source Mode  (0: Voltage)"=w488, "error in (no error)"=w491, "Output Level (0)"=w487, "VISA resource name"=w490) -> ("error out"=w495:errorcluster, "VISA resource name out"=w493:refnum<visa-resource-name>)  [unwired: 6 in]
              n84 = call "Ke2400 Enable.vi"("error in (no error)"=w495, "ON/OFF"=TRUE ("Enable Output (T: Enable)"), "VISA resource name"=w493) -> ("error out"=w492:errorcluster, "VISA resource name out"=w489:refnum<visa-resource-name>)  [unwired: 7 in]
            }
          }
          n85 = case shown="6" "Bank to HD" {
            tunnel: "070201" -> [w506 w508 w511 w514 w517 w520 w523]
            tunnel: [w504 w507 w510 w513 w516 w519 w522] -> w296
            frame 0, Default {
              n86 = Concatenate Strings(w506, "000000" ("string")) -> (w504:string)
            }
            frame 1 {
              n87 = Concatenate Strings(w508, "3B3B3B" ("string")) -> (w507:string)
            }
            frame 2 {
              n88 = Concatenate Strings(w511, "3B0000" ("string")) -> (w510:string)
            }
            frame 3 {
              n89 = Concatenate Strings(w514, "003B00" ("string")) -> (w513:string)
            }
            frame 4 {
              n90 = Concatenate Strings(w517, "00003B" ("string")) -> (w516:string)
            }
            frame 5 {
              n91 = Concatenate Strings(w520, "070707" ("string")) -> (w519:string)
            }
            frame 6 {
              n92 = Concatenate Strings(w523, "040404" ("string")) -> (w522:string)
            }
          }
          n93 = Array Max & Min(array="Set Delay") -> (max value=w286:dbl)  [unwired: 3 out]
          n94 = Divide(x=1.0, y=w286) -> (x/y=w285:dbl)
          n95 = To Unsigned Quad Integer(1:w285) -> (0:w284:u64)
          n96 = case shown="True" "HD/Cycling" {
            tunnel: [w412 w470] -> w312
            tunnel: w304 -> [w414 w457]
            tunnel: w296 -> [_ w469]
            tunnel: [w413 w468] -> w293
            tunnel: w289 -> [w409 w454]
            tunnel: w273 -> [w417 _]
            tunnel: "Set Delay" -> [w416 _]
            tunnel: w284 -> [w415 _]
            tunnel: [w411 w456] -> w278
            tunnel: "Cyc Clock Rate (Hz)" -> [w407 _]
            tunnel: w276 -> [w406 w451]
            tunnel: w275 -> [_ w450]
            frame False {
              n97 = call "WSVCAP SHL Host TL RFFE Configure.vi"("RFFE Slave Address"=w406, "Clock Rate (Hz)"=w407, "error in"=w409, "Log (T)"=FALSE) -> ("error out"=w408:errorcluster)  [unwired: 10 in, 1 out]
              n98 = while {
                tunnel: w414 -> [w437]
                tunnel: [w427] -> w413
                tunnel: [w422] -> w412
                tunnel: w408 -> [w435]
                tunnel: [w426] -> w411
                tunnel: w417 -> [w434]
                tunnel: w416 -> [w433]
                tunnel: w415 -> [w424]
                i -> [w432]
                stop <- w430 stop-if-true
                # "Target Cycles"
                n99 = To Unsigned Quad Integer(1:w437) -> (0:w436:u64)
                n100 = case shown="0" w432 {
                  tunnel: [w443 w444] -> w420
                  tunnel: w435 -> [w442 w444]
                  tunnel: w434 -> [w441 _]
                  tunnel: w433 -> [w440 _]
                  frame 0 {
                    n101 = call "WSVCAP SHL Host TL RFFE Write Cycle - Multiple DUTs - Common Data1.vi"("Data Out (Cycle Commands)"=w441, "Post Command Delay"=w440, "error in"=w442) -> ("error out"=w443:errorcluster)  [unwired: 12 in]
                  }
                  frame 1, Default {
                  }
                }
                n102 = Multiply(x=w436, y=u64 1000) -> (x*y=w426:u64)
                n103 = call "WSVCAP SHL Host TL SPI_RFFE Query Cycle Count.vi"("error in"=w420) -> ("Cycle Count"=w419:u64, "error out"=w418:errorcluster)  [unwired: 13 in]
                "Cycle Count" <- w419
                n104 = Subtract(x=w426, y=w419) -> (x-y=w425:u64)
                n105 = Greater Or Equal?(x=w419, y=w426) -> (x >= y?=w431:bool)
                n106 = Greater?(x=w425, y=w424) -> (0:w423:bool)
                n107 = case shown="True" w431 {
                  tunnel: [w446 w448] -> w428
                  tunnel: w418 -> [w446 w447]
                  tunnel: [FALSE TRUE] -> w429
                  frame False {
                  }
                  frame True {
                    n108 = call "WSVCAP SHL Host TL RFFE Stop Write Cycle.vi"("error in"=w447) -> ("error out"=w448:errorcluster)  [unwired: 14 in]
                  }
                }
                n109 = local read "Abort"() -> (w422:bool)
                n110 = Or(x=w429, y=w422) -> (x .or. y?=w430:bool)
                n111 = case shown="True" w423 {
                  tunnel: w428 -> [w438 w439]
                  tunnel: [w438 w439] -> w427
                  frame False {
                  }
                  frame True {
                  }
                }
              }
              n112 = local write "STATUS"("Parts are cycling...." ("STATUS")) -> ()
            }
            frame True {
              n113 = call "WSVCAP SHL Host TL RFFE Configure.vi"("RFFE Slave Address"=w451, "Clock Rate (Hz)"=w450, "error in"=w454, "Log (T)"=FALSE) -> ("error out"=w453:errorcluster)  [unwired: 10 in, 1 out]
              n114 = call "WSVCAP SHL Host TL RFFE Write - Multiple DUTs - Common Data.vi"("Data Out"=w469, "error in"=w453) -> ("error out"=w463:errorcluster)  [unwired: 13 in]
              n115 = call "Delay T4.vi"("milliseconds to wait"=u32 50, "error in (no error)"=w463) -> ("error out"=w460:errorcluster)  [unwired: 9 in]
              n116 = To Unsigned Quad Integer(1:w457) -> (0:w456:u64)
              n117 = for {
                tunnel: string[] ["0761", "0762", "0763"] -> [w480] mode=indexing
                tunnel: [w476] -> w459 mode=indexing
                shift-right: [w473] -> w458
                shift-left: w460 -> [w479]
                i -> [w478]
                n118 = call "WSVCAP SHL Host TL RFFE Read - Multiple DUTs - Common Data.vi"("Data Out"=w480, "error in"=w479) -> ("RFFE Data In"=w475:string[], "error out"=w472:errorcluster)  [unwired: 12 in]
                n119 = Index Array(array=w475, index=w478) -> (element=w474:string)
                n120 = call "Delay T4.vi"("milliseconds to wait"=u32 10, "error in (no error)"=w472) -> ("error out"=w473:errorcluster)  [unwired: 9 in]
                n121 = String Subset(string=w474, offset (0)=0) -> (substring=w476:string)  [unwired: 1 in]
              }
              "Verify Drivers to Stress" <- w459
              n122 = local write "STATUS"("Parts are Holding Down...." ("STATUS")) -> ()
              n123 = Multiply(x=1000.0, y=w457) -> (x*y=w466:dbl)
              n124 = Multiply(x=60.0, y=w466) -> (x*y=w467:dbl)
              n125 = event shown="[0] Timeout" {
                selector: _ -> [_ _]
                dyn-events: _ -> [_ _]
                timeout: w467 -> [_ _]
                tunnel: ["Abort" TRUE ("Abort")] -> w470
                tunnel: w458 -> [w481 w483]
                tunnel: [w481 w483] -> w468
                event Timeout {
                  n126 = event-data() -> ()  [unwired: 1 in, 2 out]
                }
                event "Abort": Value Change {
                  n127 = event-data() -> ()  [unwired: 1 in, 3 out]
                }
              }
            }
          }
          n128 = Add(x=w278, y=w321) -> (x+y=w316:u64)
          n129 = stacked-sequence {
            seq-local: [w368 _] -> [_ w386]
            seq-local: [w367 _] -> [_ w384]
            seq-local: [w366 _] -> [_ w383]
            seq-local: [w365 _] -> [_ w382]
            tunnel: [_ w400] -> w308
            tunnel: [_ w399] -> w303
            tunnel: w293 -> [w373 _]
            tunnel: w276 -> [w372 _]
            tunnel: w279 -> [w371 _]
            tunnel: [_ w382] -> w267
            tunnel: "Keep B1 Close?" -> [w364 _]
            frame #0 {
              n130 = call "WSVCAP SHL Host TL RFFE Configure.vi"("RFFE Slave Address"=w372, "Clock Rate (Hz)"=w371, "error in"=w373, "Log (T)"=FALSE) -> ("error out"=w369:errorcluster)  [unwired: 10 in, 1 out]
              n131 = case shown="True" w364 {
                tunnel: w369 -> [w377 w381]
                tunnel: [w377 w381] -> w368
                tunnel: [string[] ["00", "01", "02", "04", "08", "0C", "10", "14", "18", "1C", "20", "24", "28", "2C", "30", "34", "38", "3B", "00"] string[] ["04"]] -> w367
                tunnel: ["070201000000" ("Data Out") "070201040404" ("Data Out")] -> w366
                tunnel: [string[] ["CMin", "F1", "F2", "S1", "S2", "S3", "S4", "S5", "S6", "S7", "S8", "S9", "S10", "S11", "S12", "S13", "S14", "S14F12", "All OFF"] string[] ["S1"]] -> w365
                frame False {
                }
                frame True {
                }
              }
            }
            frame #1 {
              w385 = dbl[][] [] ("Delta CAP_T0(pF)")
              w396 = string[] [] ("CP Current(uA)")
              n132 = call "WSVCAP SHL Host TL RFFE Write - Multiple DUTs - Common Data.vi"("Data Out"=w383, "error in"=w386) -> ("error out"=w393:errorcluster)  [unwired: 13 in]
              n133 = call "Delay T4.vi"("milliseconds to wait"=u32 100, "error in (no error)"=w393) -> ("error out"=w394:errorcluster)  [unwired: 9 in]
              n134 = local write "Delta CAP_Tc(pF)"(w385) -> ()
              n135 = local write "Delta CAP_T0(pF)"(w385) -> ()
              n136 = for {
                tunnel: w384 -> [w403] mode=indexing
                tunnel: [w402] -> w399 mode=indexing
                shift-right: [w401] -> w397
                shift-left: w394 -> [w401]
                n137 = Concatenate Strings("070201" ("string"), w403, w403, w403) -> (w402:string)
              }
              n138 = local write "CAP_Value(pF)"(string[][] [] ("VSA_Value(pF)")) -> ()
              n139 = local write "CP_IDD(uA)"("" ("CP_IDD(uA)")) -> ()
              n140 = call "WS1050 16 DUT AD7747 READ.vi"("error in"=w397, "Log (T)"=FALSE, "DUT Mask Mode (All)"=WSVCAP_SHL_I2C_DUT_Mask_Mode_Enum."All") -> ("error out"=w390:errorcluster, "AD7747 Values"=→"CMin+VCAP":string[][])  [unwired: 7 in]
              n141 = local write "C1 Min_T0"(w396) -> ()
              n142 = local write "C3 Min_T0"(w396) -> ()
              n143 = local write "C2 Min_T0"(w396) -> ()
              n144 = call "Delay T4.vi"("milliseconds to wait"=u32 100, "error in (no error)"=w390) -> ("error out"=w400:errorcluster)  [unwired: 9 in]
            }
          }
          n145 = Number To Engineering String(4:w316) -> (0:w310:string)  [unwired: 3 in]
          n146 = Number To Fractional String(number="Cycle Freq(KHz)", precision (6)=i16 2) -> (F-format string=w269:string)  [unwired: 2 in]
          n147 = Number To Fractional String(number="Stress Voltage(V)", precision (6)=i16 2) -> (F-format string=w301:string)  [unwired: 2 in]
          n148 = for {
            tunnel: w308 -> [w586]
            tunnel: [w610] -> w332
            tunnel: [w593] -> w319
            tunnel: "Comment" -> [w608]
            tunnel: "Lot#" -> [w607]
            tunnel: "Wafer#" -> [w606]
            tunnel: "SN" -> [w605]
            tunnel: "File Name" -> [w604]
            tunnel: [w603] -> w333
            tunnel: w335 -> [w603]
            tunnel: [w602] -> w334
            tunnel: w313 -> [w599]
            tunnel: w312 -> [w598]
            tunnel: [w595] -> w311
            tunnel: w310 -> [w580]
            tunnel: w309 -> [w594]
            tunnel: "TMN DC\\CAP Data Log File Path" -> [w591]
            tunnel: "Test Program" -> [w590]
            tunnel: w290 -> [w584]
            tunnel: w303 -> [w588] mode=indexing
            tunnel: w302 -> [w583]
            tunnel: w267 -> [w581] mode=indexing
            tunnel: w301 -> [w582]
            tunnel: w282 -> [w574]
            tunnel: w269 -> [w572]
            tunnel: "Keep B1 Close?" -> [w569]
            i -> [w570]
            stop <- w595 stop-if-true
            n149 = case shown="1, Default" w570 {
              tunnel: [w638 w648] -> w587
              tunnel: w586 -> [w645 w648]
              tunnel: [w644 w647] -> w585
              tunnel: w584 -> [w643 w647]
              frame 0 {
                w641 = u16 0 items=["Voltage", "Current"] ("Source Mode  (0: Voltage)")
                n150 = call "Ke2400 Configure Output.vi"("Source Mode  (0: Voltage)"=w641, "error in (no error)"=w645, "Output Level (0)"=0.0, "VISA resource name"=w643) -> ("error out"=w646:errorcluster, "VISA resource name out"=w639:refnum<visa-resource-name>)  [unwired: 6 in]
                n151 = call "Ke2400 Enable.vi"("error in (no error)"=w646, "ON/OFF"=TRUE ("Enable Output (T: Enable)"), "VISA resource name"=w639) -> ("error out"=w637:errorcluster, "VISA resource name out"=w644:refnum<visa-resource-name>)  [unwired: 7 in]
                n152 = call "Delay T4.vi"("milliseconds to wait"=u32 50, "error in (no error)"=w637) -> ("error out"=w638:errorcluster)  [unwired: 9 in]
              }
              frame 1, Default {
              }
            }
            n153 = case shown="False" w569 {
              tunnel: [w613 w618] -> w609
              tunnel: w599 -> [w612 w617]
              tunnel: w570 -> [w611 _]
              frame False {
                n154 = case shown="1..3" w611 {
                  tunnel: [1 w616] -> w613
                  tunnel: w612 -> [_ w615]
                  frame 0, Default {
                  }
                  frame 1..3 {
                    n155 = Array Size(array=w615) -> (size(s)=w616:i32)
                  }
                }
              }
              frame True {
                n156 = Array Size(array=w617) -> (size(s)=w618:i32)
              }
            }
            n157 = call "WSVCAP SHL Host TL RFFE Write - Multiple DUTs - Common Data.vi"("Data Out"=w588, "error in"=w587) -> ("error out"=w589:errorcluster)  [unwired: 13 in]
            n158 = call "Delay T4.vi"("milliseconds to wait"=u32 1, "error in (no error)"=w589) -> ("error out"=w601:errorcluster)  [unwired: 9 in]
            n159 = for {
              N: w609 -> [_]
              tunnel: w599 -> [w703]
              tunnel: w591 -> [w693]
              tunnel: [w702] -> w578
              tunnel: w601 -> [w701]
              tunnel: [w697] -> w610
              tunnel: w608 -> [w680]
              tunnel: w607 -> [w687]
              tunnel: w606 -> [w686]
              tunnel: w605 -> [w685]
              tunnel: w604 -> [w684]
              tunnel: w581 -> [w683]
              tunnel: [w678] -> w602
              tunnel: w585 -> [w670]
              tunnel: w598 -> [w669]
              tunnel: [w666] -> w596
              tunnel: w594 -> [w664]
              tunnel: w590 -> [w663]
              tunnel: w583 -> [w662]
              tunnel: w582 -> [w661]
              tunnel: w581 -> [w660]
              tunnel: w570 -> [w658]
              tunnel: w580 -> [w657]
              tunnel: [w655] -> w577
              tunnel: [w654] -> w576
              tunnel: [w653] -> w575
              tunnel: [w652] -> w573
              tunnel: w572 -> [w651]
              tunnel: "VSA_IDD(A)" -> [w650]
              tunnel: w569 -> [w649]
              i -> [w656]
              stop <- w666 stop-if-true
              n160 = flat-sequence {
                tunnel: w703 -> [w761]
                tunnel: w656 -> [w760]
                tunnel: w701 -> [w762]
                tunnel: [w730] -> w698
                tunnel: [w743] -> w696
                tunnel: [w744] -> w695
                tunnel: [w745] -> w694
                tunnel: [w716] -> w692
                tunnel: [w706] -> w691
                tunnel: [w742] -> w690
                tunnel: [w741] -> w689
                tunnel: [w740] -> w688
                tunnel: w683 -> [w739]
                tunnel: [w739] -> w682
                tunnel: [w738] -> w681
                tunnel: w680 -> [w738]
                tunnel: [w710] -> w679
                tunnel: [w737] -> w676
                tunnel: [w736] -> w675
                tunnel: [w735] -> w674
                tunnel: [w725] -> w673
                tunnel: [w724] -> w672
                tunnel: [w723] -> w671
                tunnel: w670 -> [w722]
                tunnel: w669 -> [w721]
                tunnel: [w721] -> w668
                tunnel: [w720] -> w665
                tunnel: w664 -> [w720]
                tunnel: w658 -> [w718]
                tunnel: w662 -> [w711]
                tunnel: w660 -> [w717]
                tunnel: w658 -> [w715]
                tunnel: [w715] -> w659
                tunnel: w656 -> [w714]
                tunnel: w650 -> [w705]
                tunnel: w649 -> [w704]
                tunnel: [w878] -> w699
                tunnel: [w880] -> w697
                tunnel: [w879] -> w678
                tunnel: [w877] -> w655
                tunnel: [w876] -> w654
                tunnel: [w875] -> w653
                tunnel: w674 -> [w877]
                tunnel: w675 -> [w876]
                tunnel: w676 -> [w875]
                tunnel: w679 -> [w879]
                tunnel: w681 -> [w862]
                tunnel: w682 -> [w849]
                tunnel: w688 -> [w863]
                tunnel: w689 -> [w864]
                tunnel: w690 -> [w865]
                tunnel: w684 -> [w866]
                tunnel: w691 -> [w867]
                tunnel: w692 -> [w860]
                tunnel: w685 -> [w868]
                tunnel: w686 -> [w869]
                tunnel: w687 -> [w870]
                tunnel: w693 -> [w871]
                tunnel: w694 -> [w872]
                tunnel: w695 -> [w873]
                tunnel: w696 -> [w874]
                tunnel: w698 -> [w880]
                tunnel: w673 -> [w853]
                tunnel: w672 -> [w854]
                tunnel: w671 -> [w852]
                tunnel: w668 -> [w850]
                tunnel: [w850] -> w667
                tunnel: w665 -> [w848]
                tunnel: w663 -> [w847]
                tunnel: w661 -> [w846]
                tunnel: w659 -> [w845]
                tunnel: [w845] -> w652
                tunnel: w657 -> [w844]
                tunnel: w651 -> [w843]
                frame #0 {
                  w748 = FALSE ("Log (T)")
                  n161 = case shown="True" w704 {
                    tunnel: w762 -> [w773 w811]
                    tunnel: w761 -> [w772 w807]
                    tunnel: w760 -> [w771 w806]
                    tunnel: [w770 w809] -> w730
                    tunnel: w722 -> [w769 w810]
                    tunnel: [w768 w801] -> w719
                    tunnel: w718 -> [w767 _]
                    tunnel: w717 -> [w766 w802]
                    tunnel: [w765 w803] -> w716
                    tunnel: [w764 w808] -> w709
                    tunnel: w705 -> [w763 w800]
                    frame False {
                      n162 = case shown="1..3" w767 {
                        tunnel: w773 -> [w792 w797]
                        tunnel: w772 -> [w791 _]
                        tunnel: w771 -> [w790 _]
                        tunnel: [w775 w797] -> w764
                        tunnel: [w783 w796] -> w770
                        tunnel: w769 -> [w782 w796]
                        tunnel: [w778 "0"] -> w765
                        tunnel: [w777 w793] -> w768
                        tunnel: w766 -> [w776 w794]
                        tunnel: w763 -> [w774 _]
                        frame 1..3 {
                          w784 = u16 0 items=["Voltage", "Current"] ("Source Mode  (0: Voltage)")
                          n163 = Index Array(array=w791, index=w790) -> (element=w780:dbl)
                          n164 = call "Ke2400 Configure Output.vi"("Source Mode  (0: Voltage)"=w784, "error in (no error)"=w792, "Compliance  Level (0.1)"=w774, "Output Level (0)"=w780, "VISA resource name"=w782) -> ("error out"=w788:errorcluster, "VISA resource name out"=w786:refnum<visa-resource-name>)  [unwired: 5 in]
                          n165 = call "Ke2400 Enable.vi"("error in (no error)"=w788, "ON/OFF"=TRUE ("Enable Output (T: Enable)"), "VISA resource name"=w786) -> ("error out"=w789:errorcluster, "VISA resource name out"=w783:refnum<visa-resource-name>)  [unwired: 7 in]
                          n166 = Number To Fractional String(number=w780, precision (6)=i16 2) -> (F-format string=w778:string)  [unwired: 2 in]
                          n167 = call "Delay T4.vi"("milliseconds to wait"=u32 50, "error in (no error)"=w789) -> ("error out"=w775:errorcluster)  [unwired: 9 in]
                          n168 = Concatenate Strings(w776, "_Sweeping Voltage on CAP Head... ", w778) -> (w777:string)
                        }
                        frame 0, Default {
                          n169 = Concatenate Strings(w794, "_No Sweeping Voltage on CAP Head... ") -> (w793:string)
                        }
                      }
                    }
                    frame True {
                      w812 = u16 0 items=["Voltage", "Current"] ("Source Mode  (0: Voltage)")
                      n170 = Index Array(array=w807, index=w806) -> (element=w799:dbl)
                      n171 = call "Ke2400 Configure Output.vi"("Source Mode  (0: Voltage)"=w812, "error in (no error)"=w811, "Compliance  Level (0.1)"=w800, "Output Level (0)"=w799, "VISA resource name"=w810) -> ("error out"=w816:errorcluster, "VISA resource name out"=w814:refnum<visa-resource-name>)  [unwired: 5 in]
                      n172 = call "Ke2400 Enable.vi"("error in (no error)"=w816, "ON/OFF"=TRUE ("Enable Output (T: Enable)"), "VISA resource name"=w814) -> ("error out"=w817:errorcluster, "VISA resource name out"=w809:refnum<visa-resource-name>)  [unwired: 7 in]
                      n173 = Number To Fractional String(number=w799, precision (6)=i16 2) -> (F-format string=w803:string)  [unwired: 2 in]
                      n174 = call "Delay T4.vi"("milliseconds to wait"=u32 50, "error in (no error)"=w817) -> ("error out"=w808:errorcluster)  [unwired: 9 in]
                      n175 = Concatenate Strings(w802, "_Sweeping Voltage on CAP Head... ", w803) -> (w801:string)
                    }
                  }
                  n176 = call "Ke2000 Reading MilAmp.vi"("error in (no error)"=w709, "VISA resource name"=w711) -> ("error out"=w708:errorcluster, "uA"=w712:string, "VISA resource name out"=w710:refnum<visa-resource-name>)  [unwired: 7 in]
                  "CP_IDD(uA)" <- w712
                  n177 = for {
                    N: 16 -> [_]
                    tunnel: w712 -> [w819]
                    tunnel: [w819] -> w706 mode=indexing
                    tunnel: w708 -> [w818]
                    tunnel: [w818] -> w707
                  }
                  n178 = local write "STATUS"(w719) -> ()
                  n179 = call "WS1050 16 DUT AD7747 READ.vi"("error in"=w707, "Log (T)"=w748, "DUT Mask Mode (All)"=WSVCAP_SHL_I2C_DUT_Mask_Mode_Enum."C1") -> ("error out"=w757:errorcluster, "AD7747 Values"=w759:string[][])  [unwired: 7 in]
                  n180 = for {
                    tunnel: w759 -> [w841] mode=indexing
                    tunnel: [w839] -> w731 mode=indexing
                    tunnel: w757 -> [w840]
                    tunnel: [w840] -> w756
                    n181 = Index Array(array=w841, index=1) -> (element=w839:string)
                  }
                  n182 = call "WS1050 16 DUT AD7747 READ.vi"("error in"=w756, "Log (T)"=w748, "DUT Mask Mode (All)"=WSVCAP_SHL_I2C_DUT_Mask_Mode_Enum."C2") -> ("error out"=w754:errorcluster, "AD7747 Values"=w753:string[][])  [unwired: 7 in]
                  n183 = for {
                    tunnel: w753 -> [w837] mode=indexing
                    tunnel: [w835] -> w732 mode=indexing
                    tunnel: w754 -> [w836]
                    tunnel: [w836] -> w752
                    n184 = Index Array(array=w837, index=3) -> (element=w835:string)
                  }
                  n185 = call "WS1050 16 DUT AD7747 READ.vi"("error in"=w752, "Log (T)"=w748, "DUT Mask Mode (All)"=WSVCAP_SHL_I2C_DUT_Mask_Mode_Enum."C3") -> ("error out"=w750:errorcluster, "AD7747 Values"=w749:string[][])  [unwired: 7 in]
                  n186 = for {
                    tunnel: w749 -> [w833] mode=indexing
                    tunnel: [w831] -> w746 mode=indexing
                    tunnel: w750 -> [w832]
                    tunnel: [w832] -> w747
                    n187 = Index Array(array=w833, index=5) -> (element=w831:string)
                  }
                  n188 = case shown="0" w714 {
                    tunnel: w747 -> [w823 w830]
                    tunnel: [w823 w830] -> w726
                    tunnel: w746 -> [w820 w827]
                    tunnel: w732 -> [w821 w828]
                    tunnel: w731 -> [w822 w829]
                    tunnel: [w822 w829] -> w743
                    tunnel: [w821 w828] -> w744
                    tunnel: [w820 w827] -> w745
                    tunnel: [w820 w826] -> w729
                    tunnel: [w821 w825] -> w728
                    tunnel: [w822 w824] -> w727
                    frame 0 {
                      "C3 Min_T0" <- w820
                      "C2 Min_T0" <- w821
                      "C1 Min_T0" <- w822
                    }
                    frame 1, Default {
                      n189 = local read "C3 Min_T0"() -> (w826:string[])
                      n190 = local read "C1 Min_T0"() -> (w824:string[])
                      n191 = local read "C2 Min_T0"() -> (w825:string[])
                    }
                  }
                  n192 = Build Array(w731, w732, w746) -> (w733:string[][])
                  n193 = Transpose 2D Array(2D array=w733) -> (transposed array=→"CAP_Value(pF)":string[][])
                  n194 = call "WS1050 VSA_Delta C Calculation.vi"("error in (no error)"=w726, "CAP_T"=w743, "CAP_T0"=w727) -> ("error out"=w725:errorcluster, 2:"Delta C(pF)"=w735:dbl[], 3:"Delta C(pF)"=w742:string[])  [unwired: 6 in]
                  n195 = call "WS1050 VSA_Delta C Calculation.vi"("error in (no error)"=w726, "CAP_T"=w744, "CAP_T0"=w728) -> ("error out"=w724:errorcluster, 2:"Delta C(pF)"=w736:dbl[], 3:"Delta C(pF)"=w741:string[])  [unwired: 6 in]
                  n196 = call "WS1050 VSA_Delta C Calculation.vi"("error in (no error)"=w726, "CAP_T"=w745, "CAP_T0"=w729) -> ("error out"=w723:errorcluster, 2:"Delta C(pF)"=w737:dbl[], 3:"Delta C(pF)"=w740:string[])  [unwired: 6 in]
                }
                frame #1 {
                  n197 = Get Date/Time In Seconds() -> (seconds since 1Jan1904=w859:timestamp)
                  n198 = Concatenate Strings(w849, w862) -> (w861:string)
                  n199 = Get Date/Time String(seconds (now)=w859, want seconds? (F)=TRUE) -> (date string=→"date string":string, time string=→"Previous Time":string)  [unwired: 1 in]
                  n200 = Merge Errors(w853, w854, w852) -> (w851:errorcluster)
                  n201 = call "WS1050_16 DUT VSA Save Data Ver1.3.vi"("TMN DC\\CAP Data Log File Path"=w871, "Lot#"=w870, "VSA_Delta C1(pF)"=w865, "Wafer#"=w869, "File Name"=w866, "VSA_Delta C2(pF)"=w864, "error in"=w851, "Comment"=w861, "CP Current(uA)"=w867, "VSA_IDD(A)"="NA", "HD Time(Min)"=w844, "Driver"=w849, "VSA_C1"=w874, "CP HD (V)"=w848, "VSA_C2"=w873, "SN"=w868, "VSA_C3"=w872, "Test Program"=w847, "Cyc_Freq(KHz)"=w843, "Voltage(V)"=w860, "Stress Voltage(V)"=w846, "VSA_Delta C3(pF)"=w863) -> ("error out"=w878:errorcluster)  [unwired: 5 in]
                }
              }
              n202 = call "Delay T4.vi"("milliseconds to wait"=u32 1, "error in (no error)"=w699) -> ("error out"=w702:errorcluster)  [unwired: 9 in]
              n203 = Unbundle By Name(w702) -> ("status"=w677:bool)
              n204 = Compound Arithmetic op=OR(w677, w667) -> (w666:bool)
            }
            n205 = case shown="17" w573 {
              tunnel: [w619 w625] -> w579
              tunnel: w578 -> [w619 w624]
              tunnel: w577 -> [_ w623]
              tunnel: w576 -> [_ w622]
              tunnel: w575 -> [_ w621]
              tunnel: w574 -> [_ w620]
              frame 0, Default {
              }
              frame 17 {
                n206 = case shown="1, Default" w620 {
                  tunnel: w623 -> [w629 w635]
                  tunnel: w622 -> [w628 w634]
                  tunnel: w621 -> [w627 w633]
                  tunnel: w624 -> [w626 w631]
                  tunnel: [w626 w631] -> w625
                  frame 0 {
                    n207 = Build Array(w629, w628, w627) -> (→"Delta CAP_T0(pF)":dbl[][])
                  }
                  frame 1, Default {
                    n208 = Build Array(w635, w634, w633) -> (→"Delta CAP_Tc(pF)":dbl[][])
                  }
                }
              }
            }
            n209 = Unbundle By Name(w578) -> ("status"=w597:bool)
            n210 = Or(x=w597, y=w596) -> (x .or. y?=w595:bool)
            n211 = call "Delay T4.vi"("milliseconds to wait"=u32 1, "error in (no error)"=w579) -> ("error out"=w593:errorcluster)  [unwired: 9 in]
          }
          n212 = flat-sequence {
            tunnel: w319 -> [w527]
            tunnel: [w527] -> w318
            tunnel: w316 -> [w525]
            tunnel: [w526] -> w317
            frame #0 {
              n213 = Greater Or Equal?(x=w525, y="Set Stress to\nComplete(Cyc/Min)") -> (x >= y?=w526:bool)
              "Stress \nCompleted(Min)" <- w525
            }
          }
          n214 = Unbundle By Name(w318) -> ("status"=w320:bool)
          n215 = call "Delay T4.vi"("milliseconds to wait"=u32 50, "error in (no error)"=w318) -> ("error out"=w331:errorcluster)  [unwired: 9 in]
          n216 = Compound Arithmetic op=OR(w317, w320, w311) -> (w299:bool)
        }
        n217 = VISA Write(VISA resource name=w246, write buffer="SOUR:FUNC VOLT;VOLT:MODE FIX;RANG 100;LEV 0.0;:SENS:FUNC \"CURR\";CURR:PROT 60E-3;RANG 100E-3;:OUTP ON", error in (no error)=w237) -> (VISA resource name out=w250:refnum<visa-resource-name>, error out=w241:errorcluster)  [unwired: 1 out]
        n218 = for {
          tunnel: w240 -> [w264]
          tunnel: w242 -> [w261] mode=indexing
          shift-right: [w259] -> w236
          shift-left: w241 -> [w265]
          tunnel: [w257] -> w239
          n219 = call "E3631A_Voltage Controller updated.vi"("VISA resource name"=w264, "I_VDD(A)"=0.2, "Channel Controller"=w261, "Voltage 1"=0.0, "Voltage 2"=3.3, "error in (no error)"=w265, "Voltage 3"=-3.3) -> ("VISA resource name out"=w257:refnum<visa-resource-name>, "error out"=w260:errorcluster)  [unwired: 7 in]
          n220 = call "Delay T4.vi"("milliseconds to wait"=u32 100, "error in (no error)"=w260) -> ("error out"=w259:errorcluster)  [unwired: 9 in]
        }
        n221 = flat-sequence {
          tunnel: w236 -> [w881]
          tunnel: [w881] -> w235
          frame #0 {
            n222 = One Button Dialog(message="Test Completed") -> ()  [unwired: 1 in, 1 out]
          }
        }
      }
      frame True {
        w883 = FALSE
      }
    }
    n223 = Wait Until Next ms Multiple(millisecond multiple=u32 100) -> ()  [unwired: 1 out]
    n224 = local write "Abort"(w57) -> ()
    n225 = local write "stop"(w58) -> ()
    n226 = Unbundle By Name(w60) -> ("status"=w75:bool)
    n227 = Compound Arithmetic op=OR(w53, w75, w67) -> (w74:bool)
    "STATUS" <- "Idle...." ("STATUS")
  }
  "Ke2000 Out" <- w24
  "PS1 Out" <- w23
  n228 = local write "Abort"(w8) -> ()
  n229 = local write "stop"(w8) -> ()
  n230 = case shown="True" w21 {
    tunnel: [w888 w890] -> w7
    tunnel: w15 -> [w888 w889]
    frame False {
    }
    frame True {
      n231 = flat-sequence {
        tunnel: w889 -> [w893]
        tunnel: [w892] -> w890
        frame #0 {
          n232 = local write "Online"(FALSE ("Online")) -> ()
          n233 = call "WSVCAP SHL Host TL Close.vi"("error in"=w893) -> ("error out"=w892:errorcluster)  [unwired: 14 in]
        }
      }
    }
  }
  "error out" <- w7
  n234 = VISA Write(VISA resource name=w16, write buffer="SOUR:FUNC VOLT;VOLT:MODE FIX;RANG 100;LEV 0.0;:SENS:FUNC \"CURR\";CURR:PROT 60E-3;RANG 100E-3;:OUTP OFF", error in (no error)=w15) -> (VISA resource name out=→"VISA resource name out":refnum<visa-resource-name>, error out=→"error out 2":errorcluster)  [unwired: 1 out]
